vi "GetInfoArray.vi"(8 "error in (no error)":errorcluster, 11 "Signal":T1) -> (0 "error out":errorcluster, 3 "InfoArray":string[][](array[string]))   [LabVIEW 2012]
uses:
  controls/#TD_Signal.ctl
  controls/#TD_SignalInfo.ctl
  #TD_RecordLineInfo.ctl
  #TD_SignalSpecInfo.ctl
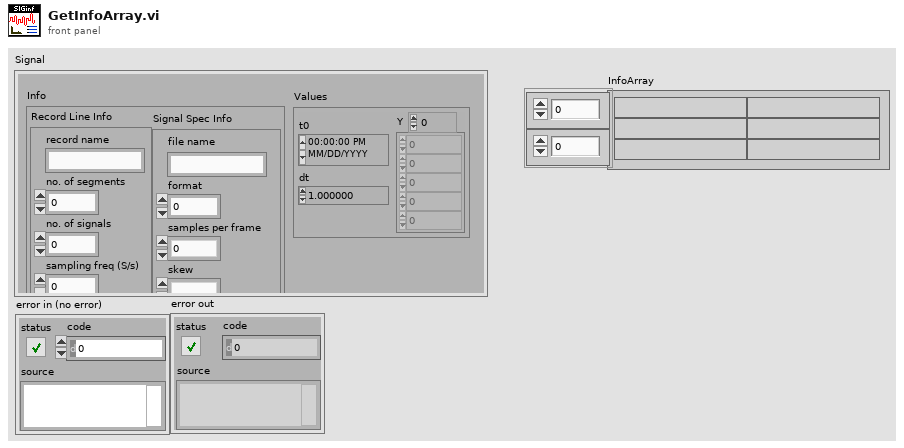
[diagram p1: front panel]
types:
  T1 = typedef "#TD_Signal.ctl" = cluster{"Info":T2, "Values":waveform(dbl)}
  T2 = typedef "#TD_SignalInfo.ctl" = cluster{"Record Line Info":T3, "Signal Spec Info":T4}
  T3 = typedef "#TD_RecordLineInfo.ctl" = cluster{"record name":string, "no. of segments":i32, "no. of signals":i32, "sampling freq (S/s)":dbl, "counter freq":dbl, "base counter value":dbl, "samples per signal":i32, "base time":string, "base date":string}
  T4 = typedef "#TD_SignalSpecInfo.ctl" = cluster{"file name":string, "format":i32, "samples per frame":i32, "skew":i32, "byte offset":i32, "ADC gain":dbl, "baseline (ADC units)":i16, "units":string, "ADC resolution":i16, "ADC zero":i16, "initial value":i16, "checksum":i16, "block size":i32, "description":string}
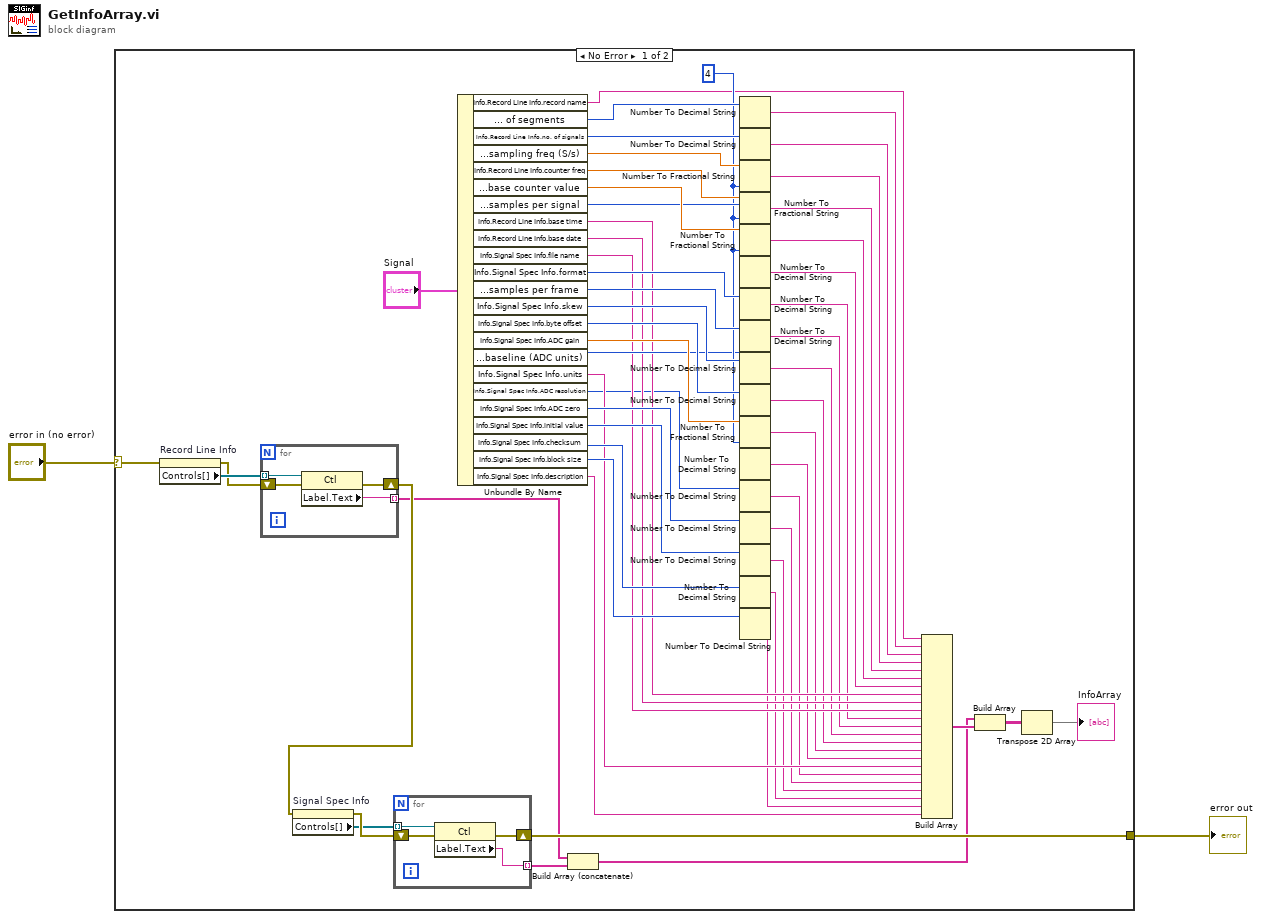
[diagram p0: block diagram]
diagram:
  n1 = case shown="No Error" "error in (no error)" {
    selector: "error in (no error)" -> [w54 w66]
    tunnel: [w50 w66] -> w1
    frame No Error {
      w36 = i16 4 ("precision (6)")
      n2 = property on="Record Line Info" class="Clust (strict)"(error in=w54) -> (error out=w53:errorcluster, "Controls[]"=w55:refnum<vi>[])  [unwired: 1 in, 1 out]
      n3 = for {
        tunnel: w55 -> [w65] mode=indexing
        tunnel: [w64] -> w49 mode=indexing
        shift-right: [w62] -> w57
        shift-left: w53 -> [w63]
        n4 = property class="Ctl"(reference=w65, error in=w63) -> (error out=w62:errorcluster, "Label.Text"=w64:string)  [unwired: 1 out]
      }
      n5 = property on="Signal Spec Info" class="Clust (strict)"(error in=w57) -> (error out=w52:errorcluster, "Controls[]"=w51:refnum<vi>[])  [unwired: 1 in, 1 out]
      n6 = for {
        tunnel: w51 -> [w61] mode=indexing
        tunnel: [w60] -> w48 mode=indexing
        shift-right: [w58] -> w50
        shift-left: w52 -> [w59]
        n7 = property class="Ctl"(reference=w61, error in=w59) -> (error out=w58:errorcluster, "Label.Text"=w60:string)  [unwired: 1 out]
      }
      n8 = Unbundle By Name("Signal") -> ("Info.Record Line Info.record name"=w30:string, "Info.Record Line Info.no. of segments"=w47:i32, "Info.Record Line Info.no. of signals"=w46:i32, "Info.Record Line Info.sampling freq (S/s)"=w45:dbl, "Info.Record Line Info.counter freq"=w44:dbl, "Info.Record Line Info.base counter value"=w43:dbl, "Info.Record Line Info.samples per signal"=w41:i32, "Info.Record Line Info.base time"=w23:string, "Info.Record Line Info.base date"=w22:string, "Info.Signal Spec Info.file name"=w21:string, "Info.Signal Spec Info.format"=w40:i32, "Info.Signal Spec Info.samples per frame"=w39:i32, "Info.Signal Spec Info.skew"=w38:i32, "Info.Signal Spec Info.byte offset"=w37:i32, "Info.Signal Spec Info.ADC gain"=w42:dbl, "Info.Signal Spec Info.baseline (ADC units)"=w35:i16, "Info.Signal Spec Info.units"=w14:string, "Info.Signal Spec Info.ADC resolution"=w7:i16, "Info.Signal Spec Info.ADC zero"=w34:i16, "Info.Signal Spec Info.initial value"=w33:i16, "Info.Signal Spec Info.checksum"=w32:i16, "Info.Signal Spec Info.block size"=w31:i32, "Info.Signal Spec Info.description"=w8:string)
      n9 = Build Array (concatenate)(w49, w48) -> (w5:string[])
      n10 = Number To Decimal String(number=w47) -> (decimal integer string=w29:string)  [unwired: 1 in]
      n11 = Number To Decimal String(number=w46) -> (decimal integer string=w28:string)  [unwired: 1 in]
      n12 = Number To Fractional String(number=w45, precision (6)=w36) -> (F-format string=w27:string)  [unwired: 2 in]
      n13 = Number To Fractional String(number=w44, precision (6)=w36) -> (F-format string=w26:string)  [unwired: 2 in]
      n14 = Number To Fractional String(number=w43, precision (6)=w36) -> (F-format string=w25:string)  [unwired: 2 in]
      n15 = Number To Decimal String(number=w41) -> (decimal integer string=w24:string)  [unwired: 1 in]
      n16 = Number To Decimal String(number=w40) -> (decimal integer string=w20:string)  [unwired: 1 in]
      n17 = Number To Decimal String(number=w39) -> (decimal integer string=w19:string)  [unwired: 1 in]
      n18 = Number To Decimal String(number=w38) -> (decimal integer string=w18:string)  [unwired: 1 in]
      n19 = Number To Decimal String(number=w37) -> (decimal integer string=w17:string)  [unwired: 1 in]
      n20 = Number To Fractional String(number=w42, precision (6)=w36) -> (F-format string=w16:string)  [unwired: 2 in]
      n21 = Number To Decimal String(number=w35) -> (decimal integer string=w15:string)  [unwired: 1 in]
      n22 = Number To Decimal String(number=w7) -> (decimal integer string=w13:string)  [unwired: 1 in]
      n23 = Number To Decimal String(number=w34) -> (decimal integer string=w12:string)  [unwired: 1 in]
      n24 = Number To Decimal String(number=w33) -> (decimal integer string=w11:string)  [unwired: 1 in]
      n25 = Number To Decimal String(number=w32) -> (decimal integer string=w10:string)  [unwired: 1 in]
      n26 = Number To Decimal String(number=w31) -> (decimal integer string=w9:string)  [unwired: 1 in]
      n27 = Build Array(w30, w29, w28, w27, w26, w25, w24, w23, w22, w21, w20, w19, w18, w17, w16, w15, w14, w13, w12, w11, w10, w9, w8) -> (w6:string[])
      n28 = Build Array(w5, w6) -> (w4:string[][])
      n29 = Transpose 2D Array(2D array=w4) -> (transposed array=→"InfoArray":string[][])
    }
    frame Error {
    }
  }
  "error out" <- w1
